vi "SetHomedState.vi"(8 "error in (no error)":errorcluster, 9 "Homing":bool, 10 "Motion Complete on all axes":bool, 11 "VXMx2 in":refnum<class "VXMx2.lvclass">) -> (0 "error out":errorcluster, 3 "VXMx2 out":refnum<class "VXMx2.lvclass">)   [LabVIEW 2019, in "VXMx2.lvclass"]
doc: "This is a space-saving VI.\nAt the end of any long motion where status is monitored, this VI checks to see if this was an establish home move, and then sets the Home Established bit = T at the end of a homing motion."
uses:
  VXMx2.lvclass
  Support/MessageAPI/UIMessage.ctl
  VXMx2.lvclass/VXMx2.ctl
  SendMessage/SendMessage.lvclass
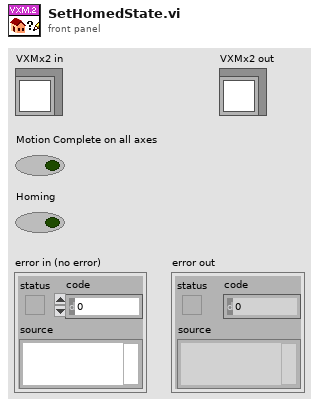
[diagram p1: front panel]
types:
  T1 = typedef "UIMessage.ctl" = cluster{"EventCode":i32, "Numeric":dbl, "String":string, "Variant":variant}
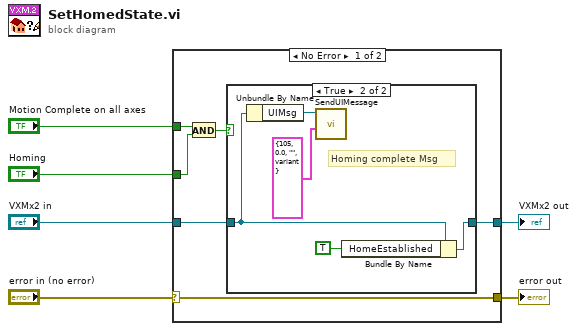
[diagram p0: block diagram]
diagram:
  n1 = case shown="No Error" "error in (no error)" {
    selector: "error in (no error)" -> [w12 w20]
    tunnel: [w12 w20] -> w1
    tunnel: [w10 w19] -> w2
    tunnel: "VXMx2 in" -> [w11 w19]
    tunnel: "Motion Complete on all axes" -> [w8 _]
    tunnel: "Homing" -> [w7 _]
    frame No Error {
      n2 = And(x=w8, y=w7) -> (x .and. y?=w9:bool)
      n3 = case shown="True" w9 {
        tunnel: w11 -> [w13 w15]
        tunnel: [w13 w18] -> w10
        frame False {
        }
        frame True {
          # "Homing complete Msg"
          n4 = Unbundle By Name(w15) -> ("UIMsg"=w14:refnum<class "SendMessage.lvclass">)
          n5 = call-dynamic "SendUIMessage.vi"("UIMsg"=T1 {"EventCode"=105, "Numeric"=0.0, "String"="", "Variant"=variant}, "SendMessage in"=w14) -> ()  [unwired: 8 in, 2 out]
          n6 = Bundle By Name(cluster=w15, "HomeEstablished"=TRUE) -> (w18:refnum<class "VXMx2.lvclass">)
        }
      }
    }
    frame Error {
    }
  }
  "error out" <- w1
  "VXMx2 out" <- w2
